vi "Configure AI Moving Average.vi"(0 "VISA resource name":refnum<visa-resource-name>, 5 "AI Channel (0001)":string="0001", 7 "Enable Moving Average (Disable)":bool, 9 "Count (2)":i32=2 min=2 max=100, 11 "error in (no error)":errorcluster) -> (4 "VISA resource name out":refnum<visa-resource-name>, 6 "AI Channel":string, 15 "error out":errorcluster)   [LabVIEW 2020, in "Yokogawa GX Series.lvlib"]
doc: "Sets the moving average of an AI channel.\n\nCommand: SMoveAve"
uses:
  <instrlib>/Yokogawa GX Series/Yokogawa GX Series.lvlib
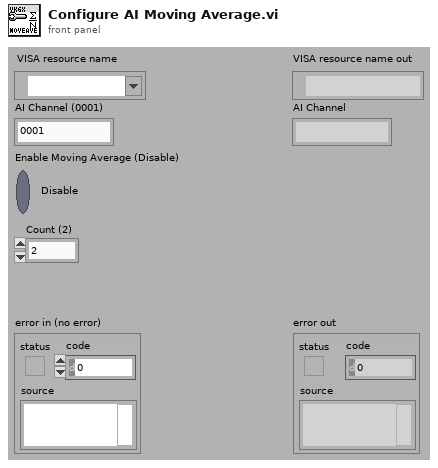
[diagram p1: front panel]
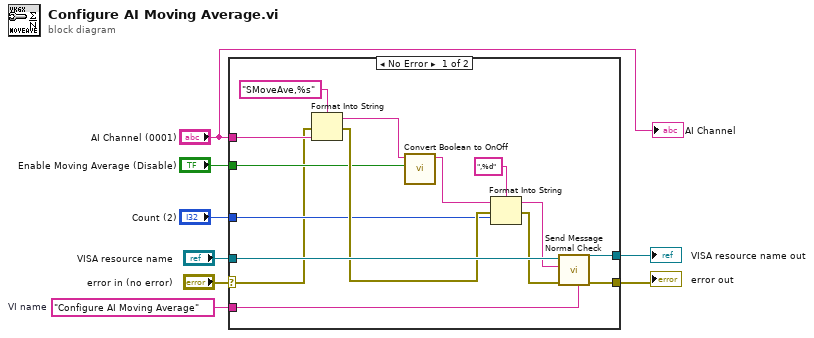
[diagram p0: block diagram]
diagram:
  w7 = "Configure AI Moving Average"  # VI name
  n1 = case shown="No Error" "error in (no error)" {
    selector: "error in (no error)" -> [w9 w24]
    tunnel: "VISA resource name" -> [w23 w25]
    tunnel: w7 -> [w22 _]
    tunnel: [w21 w25] -> w6
    tunnel: [w20 w24] -> w5
    tunnel: "Enable Moving Average (Disable)" -> [w13 _]
    tunnel: "Count (2)" -> [w11 _]
    tunnel: "AI Channel (0001)" -> [w10 _]
    frame No Error {
      n2 = Format Into String(format string="SMoveAve,%s", error in=w9, w10) -> (resulting string=w14:string, error out=w17:errorcluster)  [unwired: 1 in]
      n3 = call <instrlib>:"Convert Boolean to OnOff.vi"("On/Off"=w13, "Initial String (\"\")"=w14) -> ("Resulting String"=w12:string)  [unwired: 9 in]
      n4 = Format Into String(format string=",%d", initial string=w12, error in=w17, w11) -> (resulting string=w16:string, error out=w15:errorcluster)
      n5 = call <instrlib>:"Send Message Normal Check.vi"("Source (\"\")"=w22, "error in (no error)"=w15, "Send Message (\"\")"=w16, "VISA resource name"=w23) -> ("error out"=w20:errorcluster, "VISA resource name out"=w21:refnum<visa-resource-name>)  [unwired: 2 in, 4 out]
    }
    frame Error {
    }
  }
  "error out" <- w5
  "VISA resource name out" <- w6
  "AI Channel" <- "AI Channel (0001)"
